vi "dfd_Decide Stimulus Signal Length for Analysis.vi"(7 "#points in":i32, 8 "error in (no error)":errorcluster, 11 "filter in":T1={"mSRate_Fs"=1.0, "mSRate_Version"="1.0", "mSRate_Comments"="", "mSRate_OrgCoef"={"type"=enum."Undefined", "gain"=1.0, "coef a (k)"=[], "coef b (v)"=[]}, "mSRate_CurCoef"={"type"=enum."Undefined", "gain"=1.0, "coef a (k)"=[], "coef b (v)"=[]}, "mSRate_Quantized?"=FALSE, "mSRate_QCoef"={"type"=enum."Undefined", "gain"=1.0, "coef a (k)"=[], "coef b (v)"=[]}, "mSRate_QSettings"=[], "mSRate_Order"=0, "mSRate_Scaling"={"mSRate_ScaleByPowerOf2?"=FALSE, "mSRate_ScaleType"=enum."No Norm"}} {"mSRate_QSettings"."source" items=["Coef a/k"=0, "Coef b/v"=7, "Input"=1, "Output"=2, "Multiplicand"=3, "Product"=4, "Sum"=5, "Delay"=6, "Gain"=8]}) -> (0 "error out":errorcluster, 3 "filter out":T1={"mSRate_Fs"=1.0, "mSRate_Version"="1.0", "mSRate_Comments"="", "mSRate_OrgCoef"={"type"=enum."Undefined", "gain"=1.0, "coef a (k)"=[], "coef b (v)"=[]}, "mSRate_CurCoef"={"type"=enum."Undefined", "gain"=1.0, "coef a (k)"=[], "coef b (v)"=[]}, "mSRate_Quantized?"=FALSE, "mSRate_QCoef"={"type"=enum."Undefined", "gain"=1.0, "coef a (k)"=[], "coef b (v)"=[]}, "mSRate_QSettings"=[], "mSRate_Order"=0, "mSRate_Scaling"={"mSRate_ScaleByPowerOf2?"=FALSE, "mSRate_ScaleType"=enum."No Norm"}} {"mSRate_QSettings"."source" items=["Coef a/k"=0, "Coef b/v"=7, "Input"=1, "Output"=2, "Multiplicand"=3, "Product"=4, "Sum"=5, "Delay"=6, "Gain"=8]}, 5 "#points out":i32)   [LabVIEW 2017, in "NI_DigFilterLicensed.lvlib"]
uses:
  <vilib>/addons/Digital Filter Design/NI_DigFilterLicensed.lvlib
  <vilib>/addons/Digital Filter Design/_Objects.llb/DFD Filter Obj.ctl
  <vilib>/addons/Digital Filter Design/_Objects.llb/DFD Filter Coef.ctl
  <vilib>/addons/Digital Filter Design/_Objects.llb/DFD Filter Structure Type Selector.ctl
  <vilib>/addons/Digital Filter Design/_Objects.llb/dfd_Internal Quantization Settings.ctl
  <vilib>/addons/Digital Filter Design/_Objects.llb/dfd_Internal Quantization Srcs.ctl
  <vilib>/addons/Digital Filter Design/_Objects.llb/DFD Coef Norm Type.ctl
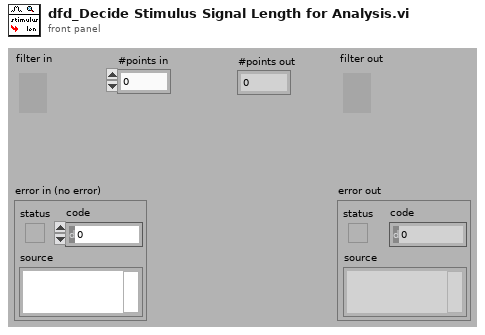
[diagram p1: front panel]
types:
  T1 = typedef "NI_DigFilterLicensed.lvlib/DFD Filter Obj.ctl" = cluster{"mSRate_Fs":dbl, "mSRate_Version":string, "mSRate_Comments":string, "mSRate_OrgCoef":T2, "mSRate_CurCoef":T2, "mSRate_Quantized?":bool, "mSRate_QCoef":T2, "mSRate_QSettings":T4[], "mSRate_Order":i32, "mSRate_Scaling":cluster{"mSRate_ScaleByPowerOf2?":bool, "mSRate_ScaleType":T6}}
  T2 = typedef "NI_DigFilterLicensed.lvlib/DFD Filter Coef.ctl" = cluster{"type":T3, "gain":dbl, "coef a (k)":dbl[], "coef b (v)":dbl[]}
  T3 = typedef "NI_DigFilterLicensed.lvlib/DFD Filter Structure Type Selector.ctl" = enum16{"Undefined", "FIR Direct Form", "FIR Direct Form Transposed", "FIR Symmetric", "FIR Antisymmetric", "IIR Direct Form I", "IIR Direct Form I Transposed", "IIR Direct Form II", "IIR Direct Form II Transposed", "IIR Cascaded Second Order Sections Form I", "IIR Cascaded Second Order Sections Form I Transposed", "IIR Cascaded Second Order Sections Form II", "IIR Cascaded Second Order Sections Form II Transposed", "Lattice Allpass (basic sections)", "Lattice Allpass (one multiplier sections)", "Lattice Allpass (normalized sections)", "Lattice AR (basic sections)", "Lattice AR (one multiplier sections)", "Lattice AR (normalized sections)", "Lattice MA (minimum phase)", "Lattice MA (maximum phase)", "Lattice ARMA (basic sections)", "Lattice ARMA (one multiplier sections)", "Lattice ARMA (normalized sections)"}
  T4 = typedef "NI_DigFilterLicensed.lvlib/dfd_Internal Quantization Settings.ctl" = cluster{"source":T5, "wl":i16, "iwl":i16, "overflow mode":enum16{"Saturation", "Wrap"}, "rounding mode":enum16{"Nearest", "Truncation"}, "signed?":bool}
  T5 = typedef "NI_DigFilterLicensed.lvlib/dfd_Internal Quantization Srcs.ctl" = u16
  T6 = typedef "NI_DigFilterLicensed.lvlib/DFD Coef Norm Type.ctl" = enum16{"No Norm", "Time Domain 1-Norm", "Time Domain 2-Norm", "Time Domain Inf-Norm"}
  T7 = typedef "NI_DigFilterLicensed.lvlib/DFD Filter Structure Id.ctl" = enum16{"Undefined", "FIR", "IIR Direct", "IIR SOS", "IIR Allpass", "IIR AR", "IIR ARMA"}
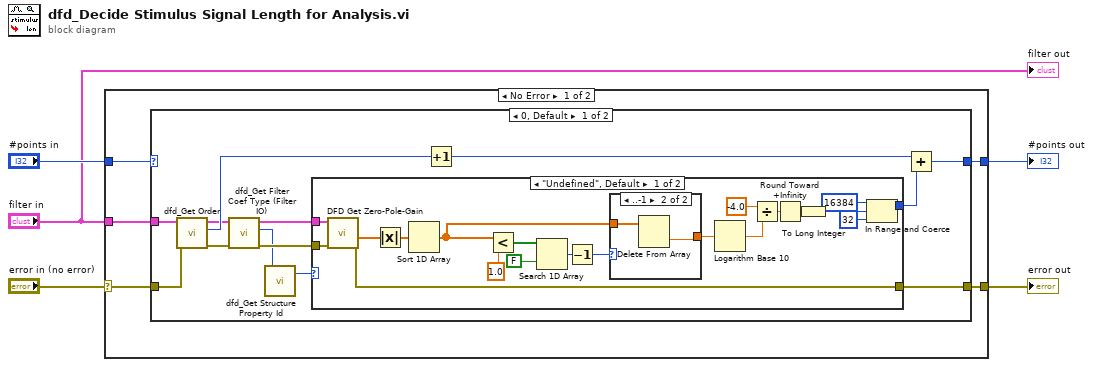
[diagram p0: block diagram]
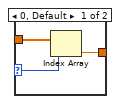
[diagram p2: hidden frame]
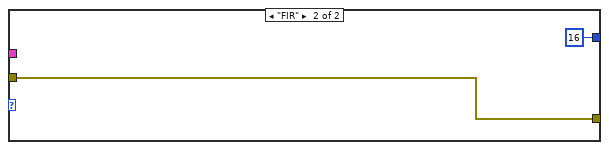
[diagram p3: hidden frame]
diagram:
  n1 = case shown="No Error" "error in (no error)" {
    selector: "error in (no error)" -> [w7 w53]
    tunnel: "#points in" -> [w10 _]
    tunnel: "filter in" -> [w8 _]
    tunnel: [w9 _] -> w2
    tunnel: [w6 w53] -> w1
    frame No Error {
      n2 = case shown="0, Default" w10 {
        selector: w10 -> [_ w52]
        tunnel: [w22 w52] -> w9
        tunnel: w8 -> [w23 _]
        tunnel: w7 -> [w21 w51]
        tunnel: [w20 w51] -> w6
        frame 0, Default {
          n3 = call <vilib>:"dfd_Get Order.vi"("error in (no error)"=w21, "filter in"=w23) -> ("error out"=w14:errorcluster, "order"=w18:i32, "filter out"=w16:T1)  [unwired: 7 out]
          n4 = call <vilib>:"dfd_Get Filter Coef Type (Filter IO).vi"("error in (no error)"=w14, "filter in"=w16) -> ("error out"=w13:errorcluster, "type"=w12:T3, "filter out"=w15:T1)  [unwired: 1 in, 6 out]
          n5 = call <vilib>:"dfd_Get Structure Property Id.vi"("structure type"=w12) -> ("filter structure id"=w11:T7)  [unwired: 1 out]
          n6 = case shown="\"Undefined\", Default" w11 {
            tunnel: [w38 w50] -> w20
            tunnel: [w37 16 ("upper limit")] -> w19
            tunnel: w15 -> [w25 _]
            tunnel: w13 -> [w24 w50]
            frame "Undefined", Default {
              n7 = call <vilib>:"DFD Get Zero-Pole-Gain.vi"("error in (no error)"=w24, "filter in"=w25) -> ("error out"=w38:errorcluster, "poles"=w35:cdb[])  [unwired: 8 out]
              n8 = Absolute Value(x=w35) -> (abs(x)=w34:dbl[])
              n9 = Sort 1D Array(array=w34) -> (sorted array=w28:dbl[])
              n10 = Less?(x=w28, y=1.0) -> (x < y?=w32:bool[])
              n11 = Search 1D Array(1D array=w32, element=FALSE) -> (index of element=w30:i32)  [unwired: 1 out]
              n12 = Decrement(x=w30) -> (x-1=w29:i32)
              n13 = case shown="..-1" w29 {
                selector: w29 -> [w45 _]
                tunnel: w28 -> [w46 w48]
                tunnel: [w44 w47] -> w27
                frame 0, Default {
                  n14 = Index Array(array=w46, index=w45) -> (element=w44:dbl)
                }
                frame ..-1 {
                  n15 = Delete From Array(array=w48) -> (deleted portion=w47:dbl)  [unwired: 2 in, 1 out]
                }
              }
              n16 = Logarithm Base 10(1:w27) -> (0:w42:dbl)
              n17 = Divide(x=-4.0, y=w42) -> (x/y=w41:dbl)
              n18 = Round Toward +Infinity(x=w41) -> (ceil(x): smallest int >= x=w26:dbl)
              n19 = To Long Integer(number=w26) -> (32bit integer=w36:i32)
              n20 = In Range and Coerce(upper limit=16384, x=w36, lower limit=32) -> (coerced(x)=w37:i32)  [unwired: 1 out]
            }
            frame "FIR" {
            }
          }
          n21 = Increment(x=w18) -> (x+1=w17:i32)
          n22 = Add(x=w17, y=w19) -> (x+y=w22:i32)
        }
        frame 1.. {
        }
      }
    }
    frame Error {
    }
  }
  "#points out" <- w2
  "error out" <- w1
  "filter out" <- "filter in"
